vi "Generic - DO1.vi"(0 "VISA session":refnum<visa-resource-name>="MW100", 2 "Semiphore":T1, 5 "Channel_Enum":T2=1 items=["4-20_OUT", "Pres_HI1", "Pres_HI2", "Pres_LOW", "Pres_PIN", "HEATER_TOP", "HEATER_BOT", "T_Shell", "FLOWMETER", "WATT_SENSE", "WH_TICK", "Tc_1", "Tc_2", "Tc_3", "Tc_4", "Tc_5", "Tc_6", "Tc_down", "T_Shell_2", "T_Shell_3", "T_Shell_4", "RTD_IN", "RTD_OUT", "RTD_AMB", "INTF_TEMPFLO", "INTF_READY", "INTF_START", "INTF_STOP", "DRM_LOW", "DRM_HIGH", "PWR_MAIN", "VLV_DUMP", "VLV_OUT", "VLV_IN", "WATT_HOURS", "FLOW(SAMPLE)", "GALLONS", "FLOW(GPM)", "FLOW_CALC_GAIN", "FLOW_CALC_OFFSET", "FLOW_CALC_THRESHOLD", "VLV_DUMP_2", "VLV_OUT_2", "VLV_IN_2", "VLV_DUMP_3", "VLV_OUT_3", "VLV_IN_3", "VLV_DUMP_4", "VLV_OUT_4", "VLV_IN_4", "CHAN_34", "CHAN_35", "CHAN_36"], 7 "Relay Status (0:CLOSED)":enum8{"CLOSED", "OPEN"}(ring), 11 "Error In":errorcluster) -> (4 "dup VISA session":refnum<visa-resource-name>, 15 "error out":errorcluster)   [LabVIEW 2012]
uses:
  ChannelSettings.ctl
panel:
  out "Local?":bool
  # "PWR_MAIN: CLOSED = POWER OFF"
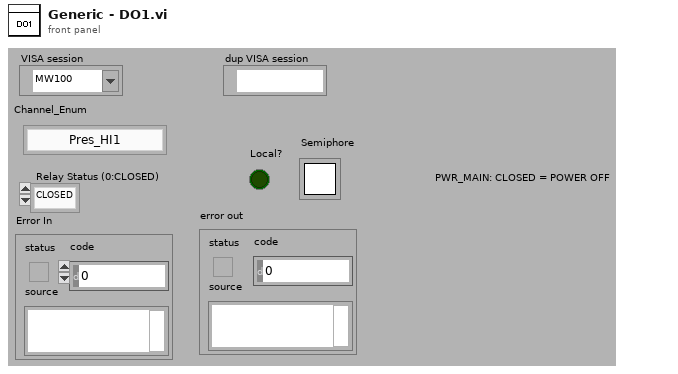
[diagram p1: front panel]
types:
  T1 = typedef "Semaphore RefNum" = refnum<k1>
  T2 = typedef "ChannelSettings.ctl" = u32
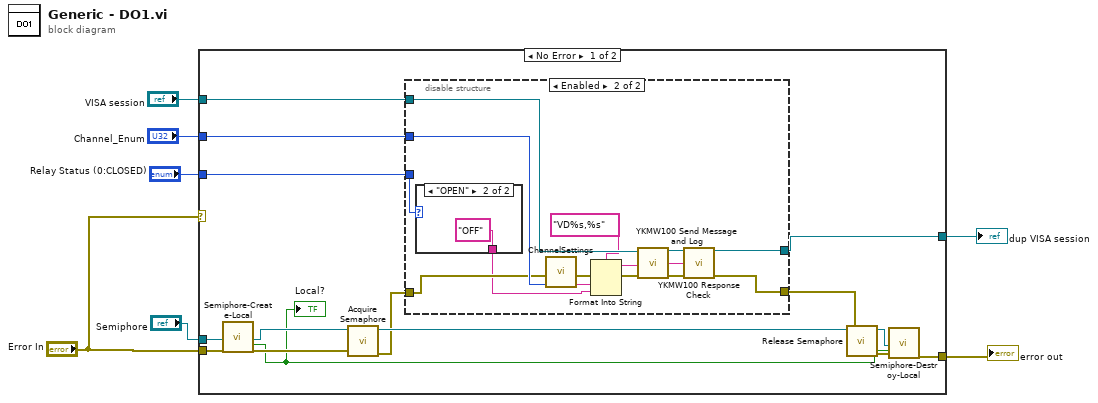
[diagram p0: block diagram]
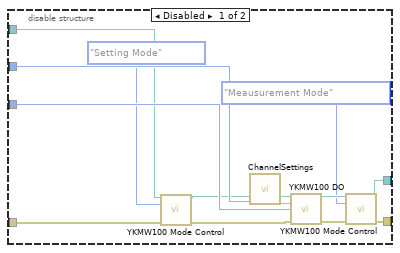
[diagram p2: hidden frame]
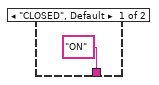
[diagram p3: hidden frame]
diagram:
  n1 = case shown="No Error" "Error In" {
    selector: "Error In" -> [_ w53]
    tunnel: "Relay Status (0:CLOSED)" -> [w22 _]
    tunnel: "Channel_Enum" -> [w21 _]
    tunnel: "VISA session" -> [w18 w52]
    tunnel: [w17 w52] -> w4
    tunnel: "Error In" -> [w15 _]
    tunnel: "Semiphore" -> [w13 _]
    tunnel: [w10 w53] -> w2
    frame No Error {
      n2 = call "Semiphore-Create-Local.vi"("Semiphore"=w13, "error in (no error)"=w15) -> ("semaphore"=w12:T1, "Local?"=w8:bool, "error out"=w14:errorcluster)  [unwired: 15 in]
      "Local?" <- w8
      n3 = call <vilib>:"Acquire Semaphore.vi"("error in (no error)"=w14, "semaphore"=w12) -> ("error out"=w19:errorcluster, "semaphore out"=w20:T1)  [unwired: 3 in, 1 out]
      n4 = disable-structure shown="Enabled" {
        disable-tunnel: w22 -> [w34 w38]
        disable-tunnel: w21 -> [w33 w40]
        disable-tunnel: w19 -> [w31 w39]
        disable-tunnel: w18 -> [w30 w42]
        disable-tunnel: [w25 w44] -> w17
        disable-tunnel: [w23 w43] -> w16
        frame Disabled {
          n5 = call "YKMW100 Mode Control.vi"("VISA session"=w30, "Model"=enum16{"Meausurement Mode", "Setting Mode"}."Setting Mode", "error in (no error)"=w31) -> ("dup VISA session"=w29:refnum<visa-resource-name>, "error out"=w32:errorcluster)  [unwired: 11 in]
          n6 = call "ChannelSettings.vi"("Channel_Enum"=w33) -> ("Channel String"=w35:string)  [unwired: 10 in]
          n7 = call "YKMW100 DO.vi"("VISA session"=w29, "P1 - Channel"=w35, "Relay Status (0:CLOSED)"=w34, "error in (no error)"=w32) -> ("dup VISA session"=w26:refnum<visa-resource-name>, "error out"=w27:errorcluster)  [unwired: 10 in]
          n8 = call "YKMW100 Mode Control.vi"("VISA session"=w26, "Model"=enum16{"Meausurement Mode", "Setting Mode"}."Meausurement Mode", "error in (no error)"=w27) -> ("dup VISA session"=w25:refnum<visa-resource-name>, "error out"=w23:errorcluster)  [unwired: 11 in]
        }
        frame Enabled {
          n9 = case shown="\"OPEN\"" w38 {
            tunnel: ["ON" "OFF"] -> w37
            frame "CLOSED", Default {
            }
            frame "OPEN" {
            }
          }
          n10 = call "ChannelSettings.vi"("Channel_Enum"=w40) -> ("Channel String"=w41:string)  [unwired: 10 in]
          n11 = Format Into String(format string="VD%s,%s", error in=w39, w41, w37) -> (resulting string=w48:string, error out=w49:errorcluster)  [unwired: 1 in]
          n12 = call "YKMW100 Send Message and Log.vi"("VISA session"=w42, "Send Message (\"\")"=w48, "error in (no error)"=w49) -> ("dup VISA session"=w47:refnum<visa-resource-name>, "Read Buffer"=w45:string, "error out"=w46:errorcluster)  [unwired: 10 in]
          n13 = call "YKMW100 Response Check.vi"("VISA session"=w47, "Message In (\"\")"=w45, "error in (no error)"=w46) -> ("dup VISA session"=w44:refnum<visa-resource-name>, "error out"=w43:errorcluster)  [unwired: 8 in, 3 out]
        }
      }
      n14 = call <vilib>:"Release Semaphore.vi"("error in (no error)"=w16, "semaphore"=w20) -> ("error out"=w11:errorcluster, "semaphore out"=w9:T1)  [unwired: 4 in]
      n15 = call "Semiphore-Destroy-Local.vi"("Semiphore"=w9, "Local?"=w8, "error in (no error)"=w11) -> ("error out"=w10:errorcluster)  [unwired: 16 in]
    }
    frame Error {
    }
  }
  "dup VISA session" <- w4
  "error out" <- w2
